vi "CleanUp.vi"(0 "object in":refnum<class "TC0608.lvclass">, 5 "error in (no error)":errorcluster) -> (14 "object out":refnum<class "TC0608.lvclass">, 19 "error out":errorcluster)   [LabVIEW 2023, in "TC0608.lvclass"]
uses:
  TC0608.lvclass
  TC0608.lvclass/TC0608.ctl
  Peltier controller TC/TCxxxx/TCxxxx.lvlib
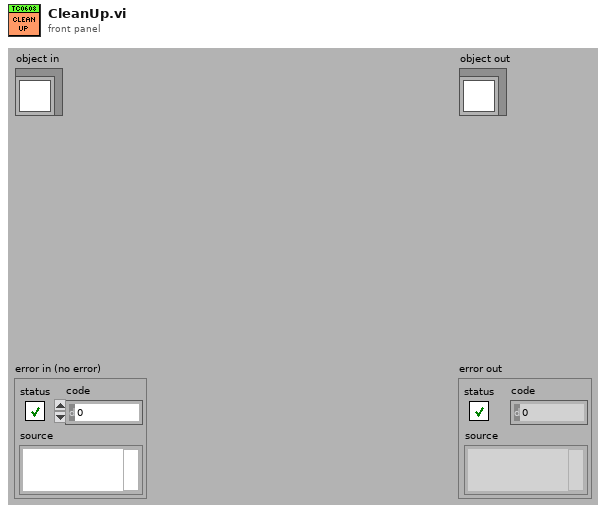
[diagram p1: front panel]
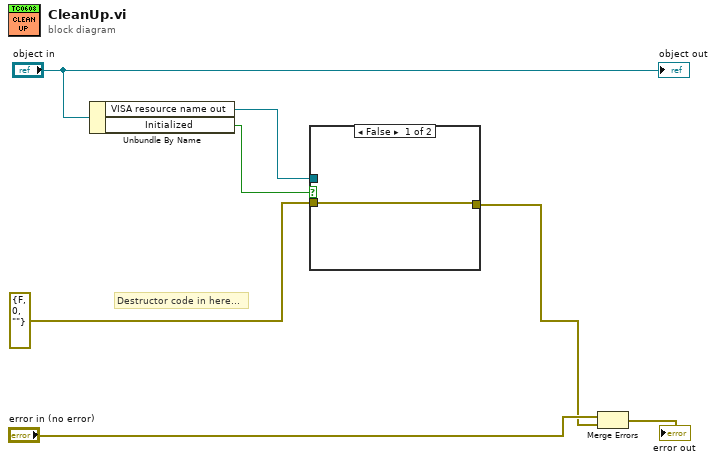
[diagram p0: block diagram]
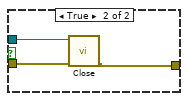
[diagram p2: hidden frame]
diagram:
  # "Destructor code in here..."
  n1 = Unbundle By Name("object in") -> ("VISA resource name out"=w4:refnum<visa-resource-name>, "Initialized"=w3:bool)
  n2 = case shown="False" w3 {
    tunnel: w4 -> [_ w11]
    tunnel: errorcluster {"status"=FALSE, "code"=0, "source"=""} ("error in (no error)") -> [w8 w10]
    tunnel: [w8 w9] -> w1
    frame False {
    }
    frame True {
      n3 = call "Close.vi"("error in (no error)"=w10, "VISA resource name"=w11) -> ("error out"=w9:errorcluster)  [unwired: 9 in]
    }
  }
  n4 = Merge Errors("error in (no error)", w1) -> (→"error out":errorcluster)
  "object out" <- "object in"
